vi "Notifier ex-1.vi"() -> ()   [LabVIEW 2022 SP3]
panel:
  out "LOOP 2":dbl
  out "loop 1":dbl
  in  "stop":bool
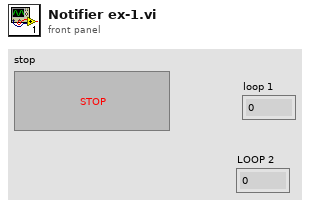
[diagram p1: front panel]
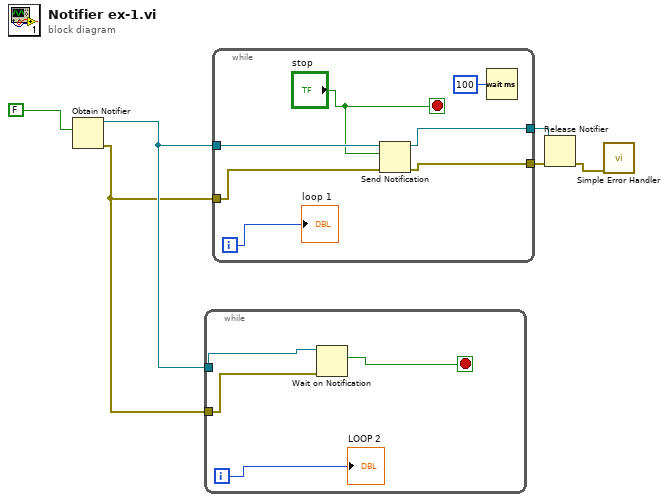
[diagram p0: block diagram]
diagram:
  n1 = Obtain Notifier(notification data type=FALSE) -> (notifier out=w5:refnum<notifier>, error out=w4:errorcluster)  [unwired: 3 in, 1 out]
  n2 = while {
    tunnel: w5 -> [w8]
    tunnel: w4 -> [w7]
    i -> [w10]
    stop <- w9 stop-if-true
    n3 = Wait on Notification(notifier=w8, error in (no error)=w7) -> (notification=w9:bool)  [unwired: 2 in, 3 out]
    "LOOP 2" <- w10
  }
  n4 = while {
    tunnel: w5 -> [w16]
    tunnel: w4 -> [w15]
    tunnel: [w12] -> w3
    tunnel: [w11] -> w2
    i -> [w17]
    stop <- "stop" stop-if-true
    n5 = Send Notification(notification="stop", notifier=w16, error in (no error)=w15) -> (notifier out=w12:refnum<notifier>, error out=w11:errorcluster)
    n6 = Wait (ms)(milliseconds to wait=u32 100) -> ()  [unwired: 1 out]
    "loop 1" <- w17
  }
  n7 = Release Notifier(notifier=w3, error in (no error)=w2) -> (error out=w1:errorcluster)  [unwired: 1 in, 2 out]
  n8 = call <vilib>:"Simple Error Handler.vi"("error in (no error)"=w1) -> ()  [unwired: 4 in, 5 out]
